vi "PS Control Server v0.80.vi"(5 "FRTZ":bool, 6 "Pause":bool, 7 "Ramp":bool, 8 "stop":bool, 9 "Slew Rate":dbl(slide)=10.0 scale=0.2..600.0 scale format="%.1f", 10 "Units":bool caption="tesla            kAmps", 11 "Setpoint":dbl format="%.2f") -> (0 "Cell":string, 1 "Status":cluster{bool, bool, "Ramp Status":u16, bool}, 2 "CurrentBar":cluster{dbl, dbl}(slide)={0.0, -0.0065359477124182705} scale=-1.0..1.0 scale format="%.1f", 3 "Current":dbl caption="Current [kA]" format="%.5f")   [LabVIEW 2021]
panel:
  out "Time(ms)":u32
  # "(To Zero Goes\nTo 100 A)"
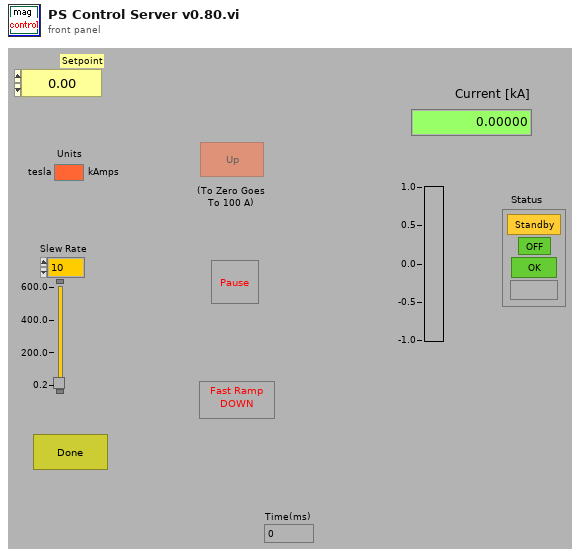
[diagram p1: front panel]
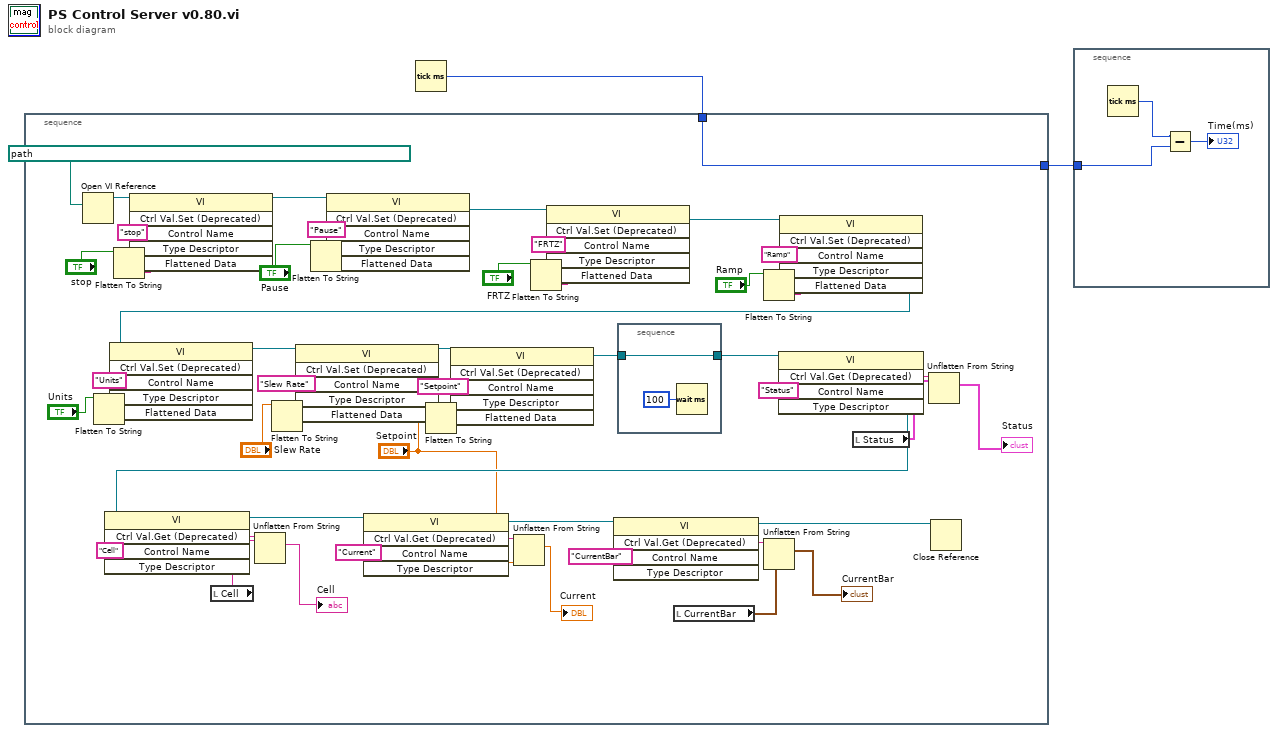
[diagram p0: block diagram]
diagram:
  n1 = Tick Count (ms)() -> (millisecond timer value=w2:u32)
  n2 = stacked-sequence {
    tunnel: [w3] -> w1
    tunnel: w2 -> [w3]
    frame #0 {
      n3 = Open VI Reference(vi path=path "/Optics2Mac/xwei Work/NML Data Acq/Serial Instruments/PS Ä/PS Control") -> (vi reference=w44:refnum<vi>)  [unwired: 5 in, 1 out]
      n4 = Flatten To String(anything="Units") -> (data string=w59:string, type string=w58:i16[])  [unwired: 3 in, 1 out]
      n5 = Flatten To String(anything="stop") -> (data string=w41:string, type string=w42:i16[])  [unwired: 3 in, 1 out]
      n6 = invoke class="VI" method="Ctrl Val.Set (Deprecated)"(reference=w44, "Control Name"="stop", "Type Descriptor"=w42, "Flattened Data"=w41) -> (reference out=w27:refnum<vi>)  [unwired: 2 in, 5 out]
      n7 = local read "Cell"() -> (w12:string)
      n8 = Flatten To String(anything="Slew Rate") -> (data string=w50:string, type string=w51:i16[])  [unwired: 3 in, 1 out]
      n9 = Flatten To String(anything="Pause") -> (data string=w29:string, type string=w30:i16[])  [unwired: 3 in, 1 out]
      n10 = invoke class="VI" method="Ctrl Val.Set (Deprecated)"(reference=w27, "Control Name"="Pause", "Type Descriptor"=w30, "Flattened Data"=w29) -> (reference out=w26:refnum<vi>)  [unwired: 2 in, 5 out]
      n11 = Flatten To String(anything="Setpoint") -> (data string=w53:string, type string=w54:i16[])  [unwired: 3 in, 1 out]
      n12 = Flatten To String(anything="FRTZ") -> (data string=w38:string, type string=w39:i16[])  [unwired: 3 in, 1 out]
      n13 = invoke class="VI" method="Ctrl Val.Set (Deprecated)"(reference=w26, "Control Name"="FRTZ", "Type Descriptor"=w39, "Flattened Data"=w38) -> (reference out=w25:refnum<vi>)  [unwired: 2 in, 5 out]
      n14 = local read "CurrentBar"() -> (w7:cluster{dbl, dbl})
      n15 = Flatten To String(anything="Ramp") -> (data string=w35:string, type string=w36:i16[])  [unwired: 3 in, 1 out]
      n16 = invoke class="VI" method="Ctrl Val.Set (Deprecated)"(reference=w25, "Control Name"="Ramp", "Type Descriptor"=w36, "Flattened Data"=w35) -> (reference out=w24:refnum<vi>)  [unwired: 2 in, 5 out]
      n17 = invoke class="VI" method="Ctrl Val.Set (Deprecated)"(reference=w24, "Control Name"="Units", "Type Descriptor"=w58, "Flattened Data"=w59) -> (reference out=w45:refnum<vi>)  [unwired: 2 in, 5 out]
      n18 = invoke class="VI" method="Ctrl Val.Set (Deprecated)"(reference=w45, "Control Name"="Slew Rate", "Type Descriptor"=w51, "Flattened Data"=w50) -> (reference out=w48:refnum<vi>)  [unwired: 2 in, 5 out]
      n19 = invoke class="VI" method="Ctrl Val.Set (Deprecated)"(reference=w48, "Control Name"="Setpoint", "Type Descriptor"=w54, "Flattened Data"=w53) -> (reference out=w16:refnum<vi>)  [unwired: 2 in, 5 out]
      n20 = stacked-sequence {
        tunnel: [w61] -> w17
        tunnel: w16 -> [w61]
        frame #0 {
          n21 = Wait (ms)(milliseconds to wait=u32 100) -> ()  [unwired: 1 out]
        }
      }
      n22 = invoke class="VI" method="Ctrl Val.Get (Deprecated)"(reference=w17, "Control Name"="Status") -> (reference out=w13:refnum<vi>, "Get Control Value"=w22:string)  [unwired: 3 in, 3 out]
      n23 = invoke class="VI" method="Ctrl Val.Get (Deprecated)"(reference=w13, "Control Name"="Cell") -> (reference out=w6:refnum<vi>, "Get Control Value"=w46:string)  [unwired: 3 in, 3 out]
      n24 = Unflatten From String(type=w12, binary string=w46) -> (value=→"Cell":string)  [unwired: 3 in, 2 out]
      n25 = invoke class="VI" method="Ctrl Val.Get (Deprecated)"(reference=w6, "Control Name"="Current") -> (reference out=w5:refnum<vi>, "Get Control Value"=w20:string)  [unwired: 3 in, 3 out]
      n26 = Unflatten From String(type="Setpoint", binary string=w20) -> (value=→"Current":dbl)  [unwired: 3 in, 2 out]
      n27 = invoke class="VI" method="Ctrl Val.Get (Deprecated)"(reference=w5, "Control Name"="CurrentBar") -> (reference out=w4:refnum<vi>, "Get Control Value"=w18:string)  [unwired: 3 in, 3 out]
      n28 = Unflatten From String(type=w7, binary string=w18) -> (value=→"CurrentBar":cluster{dbl, dbl})  [unwired: 3 in, 2 out]
      n29 = local read "Status"() -> (w15:cluster{bool, bool, "Ramp Status":u16, bool})
      n30 = Unflatten From String(type=w15, binary string=w22) -> (value=→"Status":cluster{bool, bool, "Ramp Status":u16, bool})  [unwired: 3 in, 2 out]
      n31 = Close Reference(reference=w4) -> ()  [unwired: 1 in, 1 out]
    }
  }
  n32 = stacked-sequence {
    tunnel: w1 -> [w64]
    frame #0 {
      n33 = Tick Count (ms)() -> (millisecond timer value=w65:u32)
      n34 = Subtract(x=w65, y=w64) -> (x-y=→"Time(ms)":u32)
    }
  }
